vi "GFITS_GetImname.vi"(11 "Database RefNum":T1) -> (2 "name":string)   [LabVIEW 2016]
uses:
  DBSHAND/private/vis/DatabaseHand_RefNum.ctl
  DBSHAND/private/vis/DatabaseHand_Element_Get(string).vi
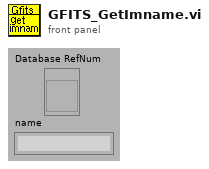
[diagram p1: front panel]
types:
  T1 = typedef "DatabaseHand_RefNum.ctl" = refnum<vi>
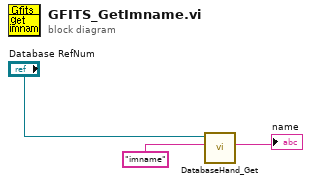
[diagram p0: block diagram]
diagram:
  n1 = call-poly "DatabaseHand_Get.vi"("name"="imname", "Database RefNum in"="Database RefNum") -> ("value"=→"name":string)  [unwired: 3 in, 6 out]
